vi "control.vi"() -> ()   [LabVIEW 2010]
panel:
  in  "Control?":bool=TRUE
  in  "Ajuste?":bool=TRUE
  in  "detla Parametros":T1
  out "Contraste":dbl
  out "Out":dbl[](array[numeric])
  in  "Parametros Maximos":T1
  in  "Sound Parameters":cluster{"# samples":u32, "tiempos (ms)":dbl}
  in  "stop":bool
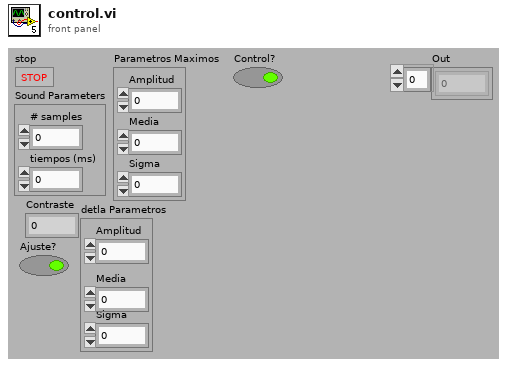
[diagram p1: front panel]
types:
  T1 = cluster{"Amplitud":dbl, "Media":dbl, "Sigma":dbl}
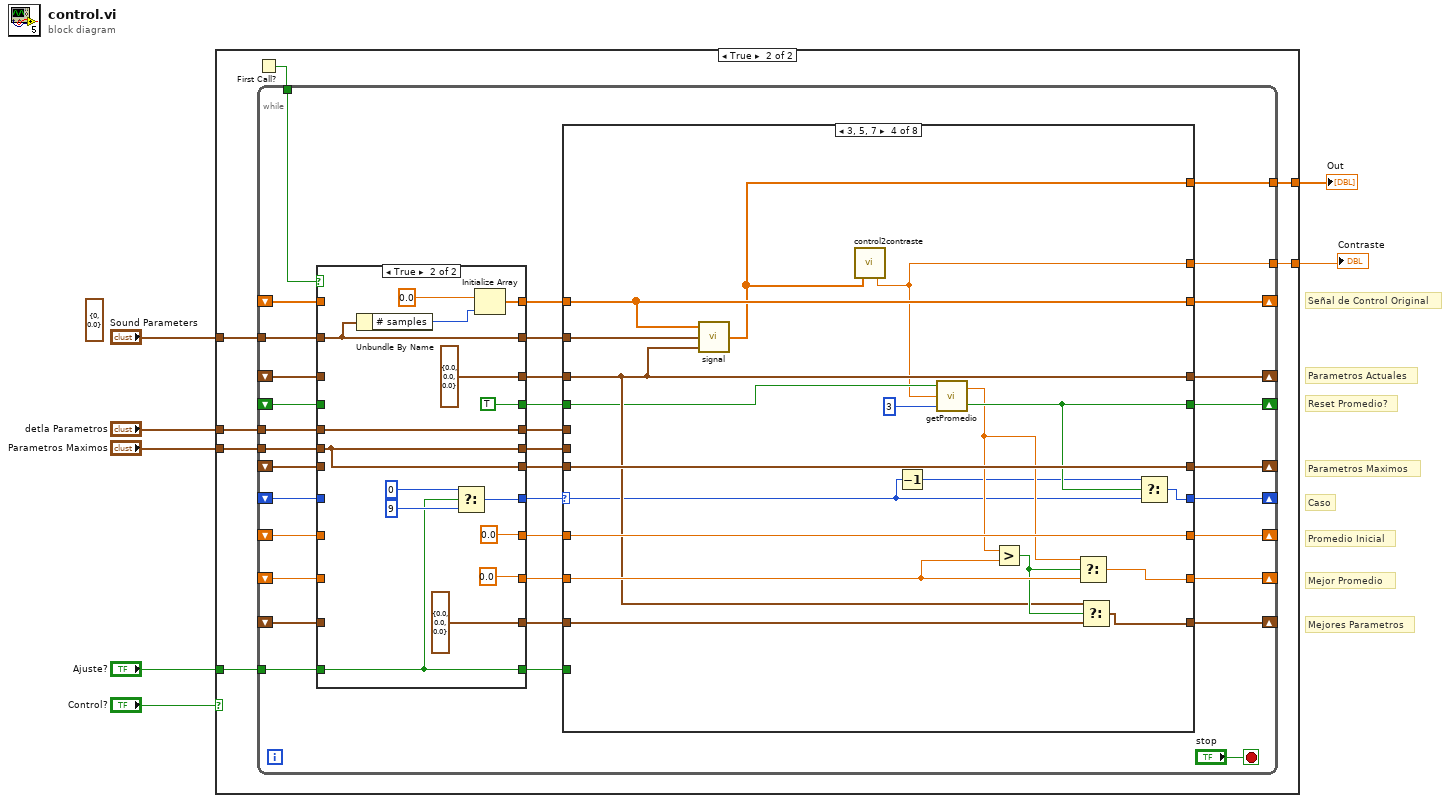
[diagram p0: block diagram]
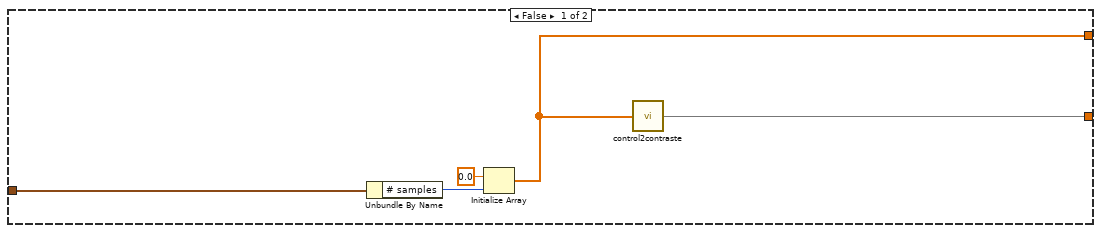
[diagram p2: hidden frame]
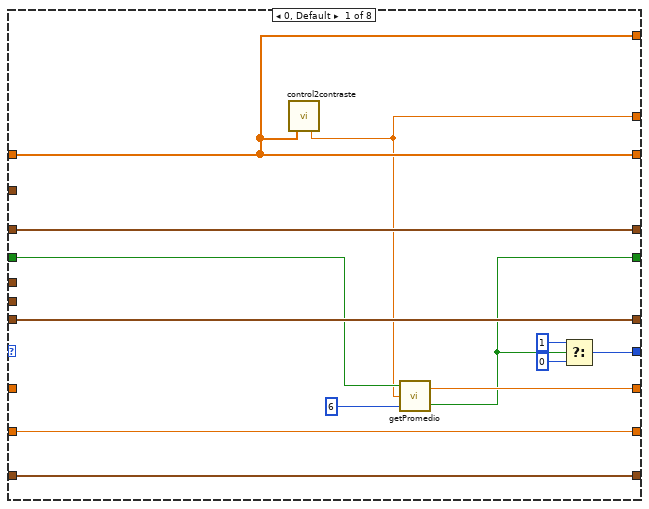
[diagram p4: hidden frame]
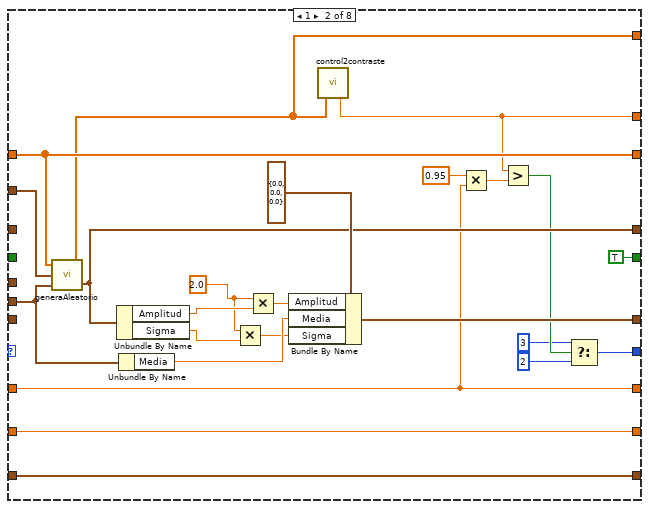
[diagram p5: hidden frame]
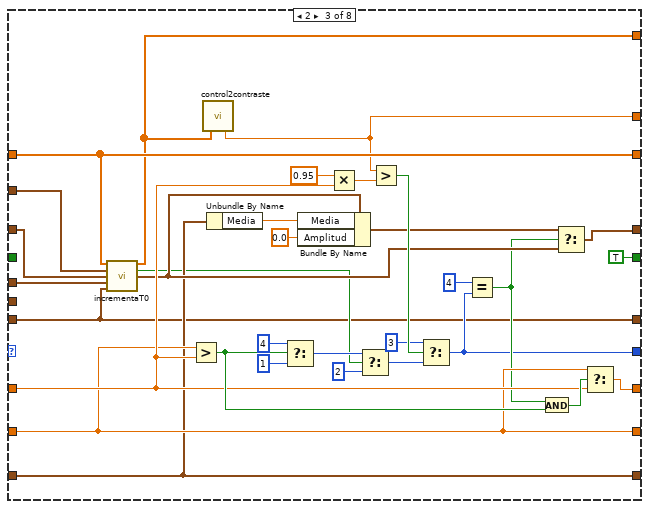
[diagram p6: hidden frame]
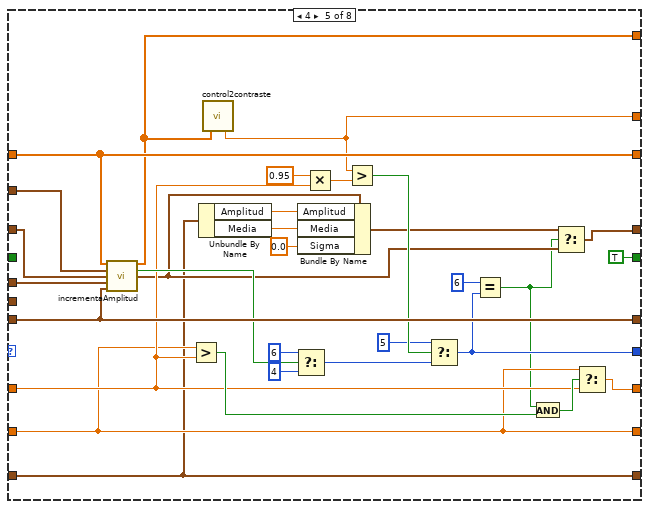
[diagram p7: hidden frame]
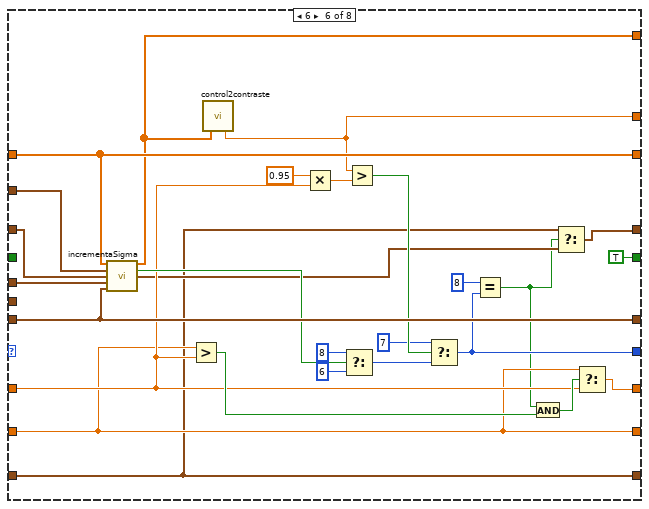
[diagram p8: hidden frame]
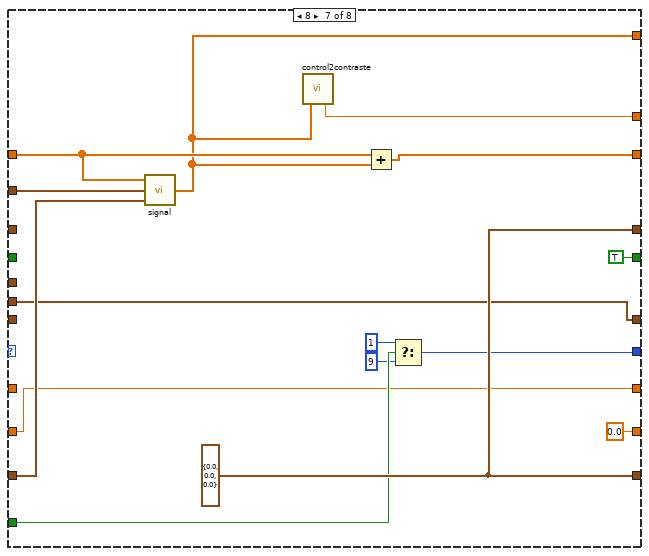
[diagram p9: hidden frame]
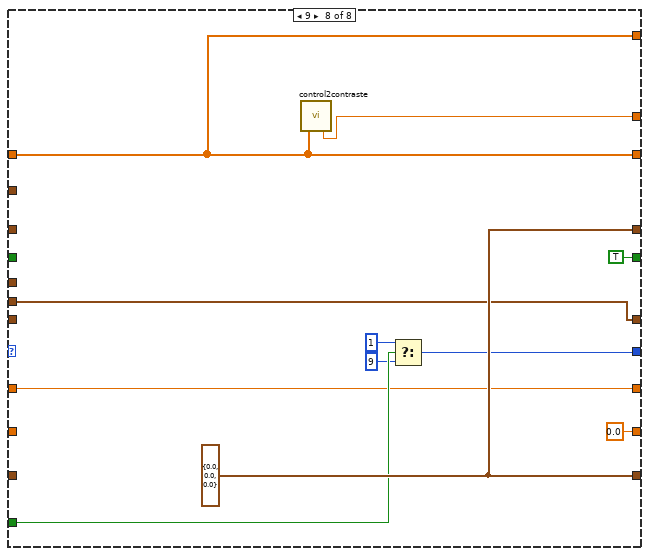
[diagram p10: hidden frame]
diagram:
  (unwired) cluster{"# samples":u32, "tiempos (ms)":dbl} {"# samples"=0, "tiempos (ms)"=0.0} ("Sound Parameters")
  # "Reset Promedio?"
  # "Mejores Parametros"
  # "Mejor Promedio"
  # "Señal de Control Original"
  # "Parametros Actuales"
  # "Parametros Maximos"
  # "Caso"
  # "Promedio Inicial"
  n1 = case shown="True" "Control?" {
    tunnel: "Sound Parameters" -> [w10 w19]
    tunnel: "detla Parametros" -> [_ w18]
    tunnel: "Parametros Maximos" -> [_ w17]
    tunnel: "Ajuste?" -> [_ w15]
    tunnel: [w8 w14] -> w2
    tunnel: [w9 w13] -> w1
    frame False {
      n2 = Unbundle By Name(w10) -> ("# samples"=w11:u32)
      n3 = Initialize Array(0.0 ("element"), w11) -> (w8:dbl[])
      n4 = call "control2contraste.vi"(1:w8) -> (0:w9)
    }
    frame True {
      n5 = First Call?() -> (First Call?: T/F=w16:bool)
      n6 = while {
        shift-right: [w51] -> _
        shift-left: _ -> [w38]
        tunnel: w19 -> [w30]
        shift-right: [w54] -> _
        shift-left: _ -> [w46]
        shift-right: [w53] -> _
        shift-left: _ -> [w40]
        shift-right: [w52] -> _
        shift-left: _ -> [w44]
        shift-right: [w50] -> _
        shift-left: _ -> [w36]
        tunnel: w18 -> [w26]
        shift-right: [w49] -> _
        shift-left: _ -> [w34]
        shift-right: [w48] -> _
        shift-left: _ -> [w32]
        shift-right: [w47] -> _
        shift-left: _ -> [w42]
        tunnel: w15 -> [w28]
        tunnel: w17 -> [w27]
        tunnel: w16 -> [w29]
        tunnel: [w21] -> w14
        tunnel: [w20] -> w13
        stop <- "stop" stop-if-true
        n7 = case shown="True" w29 {
          tunnel: w46 -> [w67 _]
          tunnel: [w67 w82] -> w45
          tunnel: [w66 T1 {"Amplitud"=0.0, "Media"=0.0, "Sigma"=0.0} ("Parametros Iniciales")] -> w43
          tunnel: w44 -> [w66 _]
          tunnel: w42 -> [w65 _]
          tunnel: [w65 TRUE] -> w41
          tunnel: w40 -> [w64 _]
          tunnel: [w64 w71] -> w39
          tunnel: w38 -> [w63 _]
          tunnel: [w63 w72] -> w37
          tunnel: w36 -> [w62 _]
          tunnel: [w62 0.0 ("Contraste Promedio")] -> w35
          tunnel: w34 -> [w61 _]
          tunnel: [w61 0.0 ("Contraste Promedio")] -> w33
          tunnel: w32 -> [w60 _]
          tunnel: [w60 T1 {"Amplitud"=0.0, "Media"=0.0, "Sigma"=0.0} ("Parametros Maximos")] -> w31
          tunnel: w30 -> [w59 w68]
          tunnel: w27 -> [w57 w71]
          tunnel: w28 -> [w56 w69]
          tunnel: [w57 w71] -> w25
          tunnel: [w58 w70] -> w24
          tunnel: w26 -> [w58 w70]
          tunnel: [w56 w69] -> w23
          tunnel: [w59 w68] -> w22
          frame False {
          }
          frame True {
            n8 = Unbundle By Name(w68) -> ("# samples"=w80:u32)
            n9 = Select(t=u32 0, s=w69, f=u32 9) -> (s? t:f=w72:u32)
            n10 = Initialize Array(0.0 ("element"), w80) -> (w82:dbl[])
          }
        }
        n11 = case shown="3, 5, 7" w37 {
          selector: w37 -> [_ _ _ w154 _ _ _ _]
          tunnel: w45 -> [w84 w118 w148 w169 w198 w225 w235 w245]
          tunnel: w22 -> [_ w119 w151 w170 w201 w228 w243 _]
          tunnel: w39 -> [w87 _ w122 w160 w197 w224 _ _]
          tunnel: [w84 w118 w148 w169 w198 w225 w234 w245] -> w54
          tunnel: [w87 w117 w122 w160 w197 w224 w231 w247] -> w53
          tunnel: [w88 w115 w131 w159 w181 w208 w240 w253] -> w52
          tunnel: [w94 w102 w123 w167 w183 w210 w232 w248] -> w51
          tunnel: [w89 w104 w137 w166 w188 w215 w233 w246] -> w50
          tunnel: w35 -> [_ w104 w135 w166 w186 w213 _ w246]
          tunnel: [w83 w96 w120 w152 w172 w202 w229 w244] -> w20
          tunnel: [w84 w97 w121 w153 w171 w203 w230 w245] -> w21
          tunnel: w43 -> [w88 _ w150 w159 w200 w227 _ _]
          tunnel: w24 -> [_ _ w149 _ w199 w226 _ _]
          tunnel: [w90 w108 w134 w165 w185 w212 0.0 ("Contraste Promedio") 0.0 ("Contraste Promedio")] -> w49
          tunnel: [w91 w107 w128 w163 w178 w204 w240 w253] -> w48
          tunnel: w31 -> [w91 w107 w128 w161 w178 w204 w242 _]
          tunnel: w33 -> [w90 w108 w134 w164 w185 w212 w233 _]
          tunnel: w41 -> [w85 _ _ w158 _ _ _ _]
          tunnel: [w86 TRUE ("Llego a N?") TRUE ("Llego a N?") w157 TRUE ("Llego a N?") TRUE ("Llego a N?") TRUE ("Llego a N?") TRUE ("Llego a N?")] -> w47
          tunnel: w23 -> [_ _ _ _ _ _ w238 w251]
          tunnel: w25 -> [_ w98 _ _ _ _ w231 w247]
          frame 0, Default {
            n12 = call "control2contraste.vi"("ControlSignal"=w84) -> ("Contraste"=w83:dbl)  [unwired: 14 in, 4 out]
            n13 = call "getPromedio.vi"("N"=6, "Contraste"=w83, "Reset"=w85) -> ("Llego a N?"=w86:bool, "Contraste Promedio"=w89:dbl)
            n14 = Select(t=u32 1, s=w86, f=u32 0) -> (s? t:f=w94:u32)
          }
          frame 1 {
            w110 = 2.0 ("x")
            n15 = call "generaAleatorio.vi"("Parametros Maximos"=w98, "Sound Parameters"=w119, "Señal de Control IN"=w118) -> ("Parametros Iniciales"=w115:T1, "Out"=w97:dbl[])
            n16 = Unbundle By Name(w115) -> ("Amplitud"=w114:dbl, "Sigma"=w111:dbl)
            n17 = Unbundle By Name(w98) -> ("Media"=w112:dbl)
            n18 = Multiply(x=w110, y=w111) -> (x*y=w109:dbl)
            n19 = Multiply(x=w110, y=w114) -> (x*y=w113:dbl)
            n20 = Bundle By Name(cluster=T1 {"Amplitud"=0.0, "Media"=0.0, "Sigma"=0.0} ("Parametros Iniciales"), "Amplitud"=w113, "Media"=w112, "Sigma"=w109) -> (w117:T1)
            n21 = call "control2contraste.vi"("ControlSignal"=w97) -> ("Contraste"=w96:dbl)  [unwired: 14 in, 4 out]
            n22 = Multiply(x=0.95, y=w104) -> (x*y=w106:dbl)
            n23 = Greater?(x=w96, y=w106) -> (0:w103:bool)
            n24 = Select(t=u32 3, s=w103, f=u32 2) -> (s? t:f=w102:u32)
          }
          frame 2 {
            n25 = call "incrementaT0.vi"("Señal de Control IN"=w148, "Sound Parameters"=w151, "Parametros Actuales IN"=w150, "detla Parametros"=w149, "Parametros Maximos"=w122) -> ("Out"=w121:dbl[], "Tope?"=w125:bool, "Parametros Actuales OUT"=w129:T1)  [unwired: 8 in]
            n26 = Greater?(x=w134, y=w135) -> (0:w138:bool)
            n27 = call "control2contraste.vi"("ControlSignal"=w121) -> ("Contraste"=w120:dbl)  [unwired: 14 in, 4 out]
            n28 = Unbundle By Name(w128) -> ("Media"=w127:dbl)
            n29 = Select(t=u32 4, s=w138, f=u32 1) -> (s? t:f=w140:u32)
            n30 = Bundle By Name(cluster=w129, "Media"=w127, "Amplitud"=0.0) -> (w130:T1)
            n31 = Multiply(x=0.95, y=w135) -> (x*y=w147:dbl)
            n32 = Select(t=w140, s=w125, f=u32 2) -> (s? t:f=w139:u32)
            n33 = Greater?(x=w120, y=w147) -> (0:w145:bool)
            n34 = Select(t=u32 3, s=w145, f=w139) -> (s? t:f=w123:u32)
            n35 = Equal?(x=u32 4, y=w123) -> (x = y?=w124:bool)
            n36 = And(x=w124, y=w138) -> (x .and. y?=w136:bool)
            n37 = Select(t=w130, s=w124, f=w129) -> (s? t:f=w131:T1)
            n38 = Select(t=w134, s=w136, f=w135) -> (s? t:f=w137:dbl)
          }
          frame 3, 5, 7 {
            n39 = call "signal.vi"("Parametros Actuales IN"=w159, "Sound Parameters"=w170, "Señal de Control IN"=w169) -> ("Out"=w153:dbl[])
            n40 = call "control2contraste.vi"("ControlSignal"=w153) -> ("Contraste"=w152:dbl)  [unwired: 14 in, 4 out]
            n41 = Decrement(x=w154) -> (x-1=w155:u32)
            n42 = call "getPromedio.vi"("N"=3, "Contraste"=w152, "Reset"=w158) -> ("Llego a N?"=w157:bool, "Contraste Promedio"=w156:dbl)
            n43 = Greater?(x=w156, y=w164) -> (0:w162:bool)
            n44 = Select(t=w156, s=w162, f=w164) -> (s? t:f=w165:dbl)
            n45 = Select(t=w159, s=w162, f=w161) -> (s? t:f=w163:T1)
            n46 = Select(t=w155, s=w157, f=w154) -> (s? t:f=w167:u32)
          }
          frame 4 {
            n47 = call "incrementaAmplitud.vi"("Señal de Control IN"=w198, "Sound Parameters"=w201, "Parametros Actuales IN"=w200, "detla Parametros"=w199, "Parametros Maximos"=w197) -> ("Out"=w171:dbl[], "Tope?"=w190:bool, "Parametros Actuales OUT"=w179:T1)  [unwired: 8 in]
            n48 = Greater?(x=w185, y=w186) -> (0:w189:bool)
            n49 = Unbundle By Name(w178) -> ("Amplitud"=w177:dbl, "Media"=w175:dbl)
            n50 = call "control2contraste.vi"("ControlSignal"=w171) -> ("Contraste"=w172:dbl)  [unwired: 14 in, 4 out]
            n51 = Select(t=u32 6, s=w190, f=u32 4) -> (s? t:f=w191:u32)
            n52 = Bundle By Name(cluster=w179, "Amplitud"=w177, "Media"=w175, "Sigma"=0.0 ("Amplitud")) -> (w180:T1)
            n53 = Multiply(x=0.95, y=w186) -> (x*y=w196:dbl)
            n54 = Greater?(x=w172, y=w196) -> (0:w194:bool)
            n55 = Select(t=u32 5, s=w194, f=w191) -> (s? t:f=w183:u32)
            n56 = Equal?(x=u32 6, y=w183) -> (x = y?=w173:bool)
            n57 = And(x=w173, y=w189) -> (x .and. y?=w187:bool)
            n58 = Select(t=w180, s=w173, f=w179) -> (s? t:f=w181:T1)
            n59 = Select(t=w185, s=w187, f=w186) -> (s? t:f=w188:dbl)
          }
          frame 6 {
            n60 = call "incrementaSigma.vi"("Señal de Control IN"=w225, "Sound Parameters"=w228, "Parametros Actuales IN"=w227, "detla Parametros"=w226, "Parametros Maximos"=w224) -> ("Out"=w203:dbl[], "Tope?"=w217:bool, "Parametros Actuales OUT"=w207:T1)  [unwired: 8 in]
            n61 = Greater?(x=w212, y=w213) -> (0:w216:bool)
            n62 = call "control2contraste.vi"("ControlSignal"=w203) -> ("Contraste"=w202:dbl)  [unwired: 14 in, 4 out]
            n63 = Multiply(x=0.95, y=w213) -> (x*y=w223:dbl)
            n64 = Select(t=u32 8, s=w217, f=u32 6) -> (s? t:f=w218:u32)
            n65 = Greater?(x=w202, y=w223) -> (0:w221:bool)
            n66 = Select(t=u32 7, s=w221, f=w218) -> (s? t:f=w210:u32)
            n67 = Equal?(x=u32 8, y=w210) -> (x = y?=w205:bool)
            n68 = And(x=w205, y=w216) -> (x .and. y?=w214:bool)
            n69 = Select(t=w204, s=w205, f=w207) -> (s? t:f=w208:T1)
            n70 = Select(t=w212, s=w214, f=w213) -> (s? t:f=w215:dbl)
          }
          frame 8 {
            w240 = T1 {"Amplitud"=0.0, "Media"=0.0, "Sigma"=0.0} ("Parametros Maximos")
            n71 = call "signal.vi"("Parametros Actuales IN"=w242, "Sound Parameters"=w243, "Señal de Control IN"=w235) -> ("Out"=w230:dbl[])
            n72 = call "control2contraste.vi"("ControlSignal"=w230) -> ("Contraste"=w229:dbl)  [unwired: 14 in, 4 out]
            n73 = Add(x=w235, y=w230) -> (x+y=w234:dbl[])
            n74 = Select(t=u32 1, s=w238, f=u32 9) -> (s? t:f=w232:u32)
          }
          frame 9 {
            w253 = T1 {"Amplitud"=0.0, "Media"=0.0, "Sigma"=0.0} ("Parametros Maximos")
            n75 = call "control2contraste.vi"("ControlSignal"=w245) -> ("Contraste"=w244:dbl)  [unwired: 14 in, 4 out]
            n76 = Select(t=u32 1, s=w251, f=u32 9) -> (s? t:f=w248:u32)
          }
        }
      }
    }
  }
  "Out" <- w2
  "Contraste" <- w1
